vi "Data File Processing UI Build File Relative Path.vi"(7 "full filename":string) -> (8 "file path out":path)   [LabVIEW 2012]
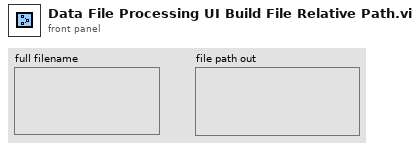
[diagram p1: front panel]
types:
  T1 = enum32{"invalid app kind", "Development System", "Run Time System", "Student Edition", "Embedded LabVIEW", "Evaluation", "Custom"}
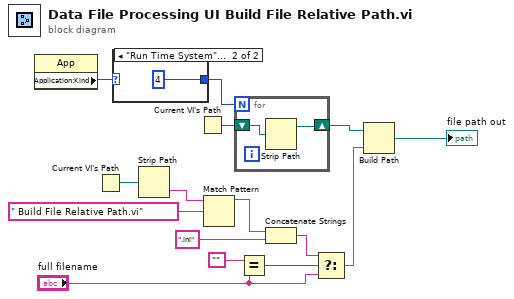
[diagram p0: block diagram]
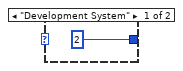
[diagram p2: hidden frame]
diagram:
  n1 = property class="App"() -> ("Application:Kind"=w15:T1)  [unwired: 2 in, 2 out]
  n2 = Current VI's Path() -> (path=w10:path)
  n3 = case shown="\"Run Time System\", Default" w15 {
    tunnel: [2 4] -> w13
    frame "Development System" {
    }
    frame "Run Time System", Default {
    }
  }
  n4 = Strip Path(path=w10) -> (name=w9:string)  [unwired: 1 out]
  n5 = Current VI's Path() -> (path=w14:path)
  n6 = Match Pattern(string=w9, regular expression=" Build File Relative Path.vi") -> (before substring=w7:string)  [unwired: 1 in, 3 out]
  n7 = for {
    N: w13 -> [_]
    shift-right: [w18] -> w12
    shift-left: w14 -> [w19]
    n8 = Strip Path(path=w19) -> (stripped path=w18:path)  [unwired: 1 out]
  }
  n9 = Equal?(x="", y="full filename") -> (x = y?=w6:bool)
  n10 = Concatenate Strings(w7, ".ini" ("string")) -> (w5:string)
  n11 = Select(t=w5, s=w6, f="full filename") -> (s? t:f=w4:string)
  n12 = Build Path(base path=w12, name or relative path=w4) -> (appended path=→"file path out":path)
